vi "Halvorsen_Basic_Methods.vi"() -> ()   [LabVIEW 2016]
uses:
  <vilib>/Simulation/Scripting/Companion Diagram/SimConfigNode/SimParams.ctl
  <vilib>/Simulation/Scripting/Companion Diagram/SimConfigNode/_simSolvers.ctl
  <vilib>/Simulation/Implementation/Shared/SIMSCR Execution Mode.ctl
  <vilib>/Simulation/Param Hierarchy/Typedefs/SIMPH Param Control Actions.ctl
  <vilib>/Simulation/Implementation/Shared/SIM limit type.ctl
  <vilib>/Simulation/Implementation/Shared/NILVSim_ParamChanged.vi
  <vilib>/Simulation/Implementation/Shared/NILVSIM_BeginStep.vi
  <vilib>/Simulation/ContinuousLinear/Implementation/NILVSim Integrator new.llb/SIM Integrator Distributor (vector).vi
  <vilib>/Simulation/Utility/Implementation/NILVSim Collector.llb/SIM Collector (scalar).vi
  <vilib>/Simulation/ContinuousLinear/Implementation/NILVSim Integrator new.llb/SIM Integrator Collector (vector).vi
  <vilib>/Simulation/Implementation/Shared/NILVSim_Manager.vi
  <vilib>/Utility/error.llb/Clear Errors.vi
  <vilib>/Simulation/Implementation/Shared/NILVSim_FinalizeModel.vi
  <vilib>/Simulation/Utility/Implementation/NILVSim Collector.llb/NILVSim Collector core (scalar).vi
  <vilib>/Simulation/Implementation/Shared/SIM Unbundle Sim Info.vi
  <vilib>/Simulation/Implementation/Shared/NILVSim_Initialize.vi
  <vilib>/Simulation/Utility/Implementation/NILVSim Get Time and IsAcceptedStep.vi
  <vilib>/Simulation/Implementation/Shared/SIMSH Read Queue.vi
  <vilib>/Simulation/Implementation/Shared/NILVSim_GetModelError.vi
  <vilib>/Simulation/Implementation/Shared/SIM Bundle Sim Info.vi
  <vilib>/Simulation/Scripting/Companion Diagram/SimConfigNode/SimDog.xnode
  <vilib>/Simulation/Implementation/XNodeFramework/SimXNode/SimX.xnode
  <vilib>/Simulation/ContinuousLinear/Implementation/NILVSim Integrator new.llb/SIM Integrator (vector).vi
  <vilib>/Simulation/Implementation/Shared/NI_SIM_Implementation.lvlib
panel:
  in  "Method Stepsize":dbl=0.01
  in  "Parameters":dbl[](array[numeric])=[0.1, 0.1, 0.1]
  in  "Method":u16=1
  out "Абсолютная погрешность":ext[][](graph)
  out "last_point_Thomas":dbl[](array[numeric])=[2.5014012033767568, 0.2778214910167161, 0.25145974992803094] format="%#_22f"
  in  "ODE Solver":T1(ring)=enum."Runge-Kutta 45 (variable)"
  out "Временная область":dbl[][](graph)
  in  "SM Step":dbl=0.005
  in  "T":dbl=100.0
  in  "Intial condition":dbl[](array[knob])=[1.0, 0.0, 1.0] scale=-10.0..10.0
  # "0,19"
  # "0,1"
  # "0,208186"
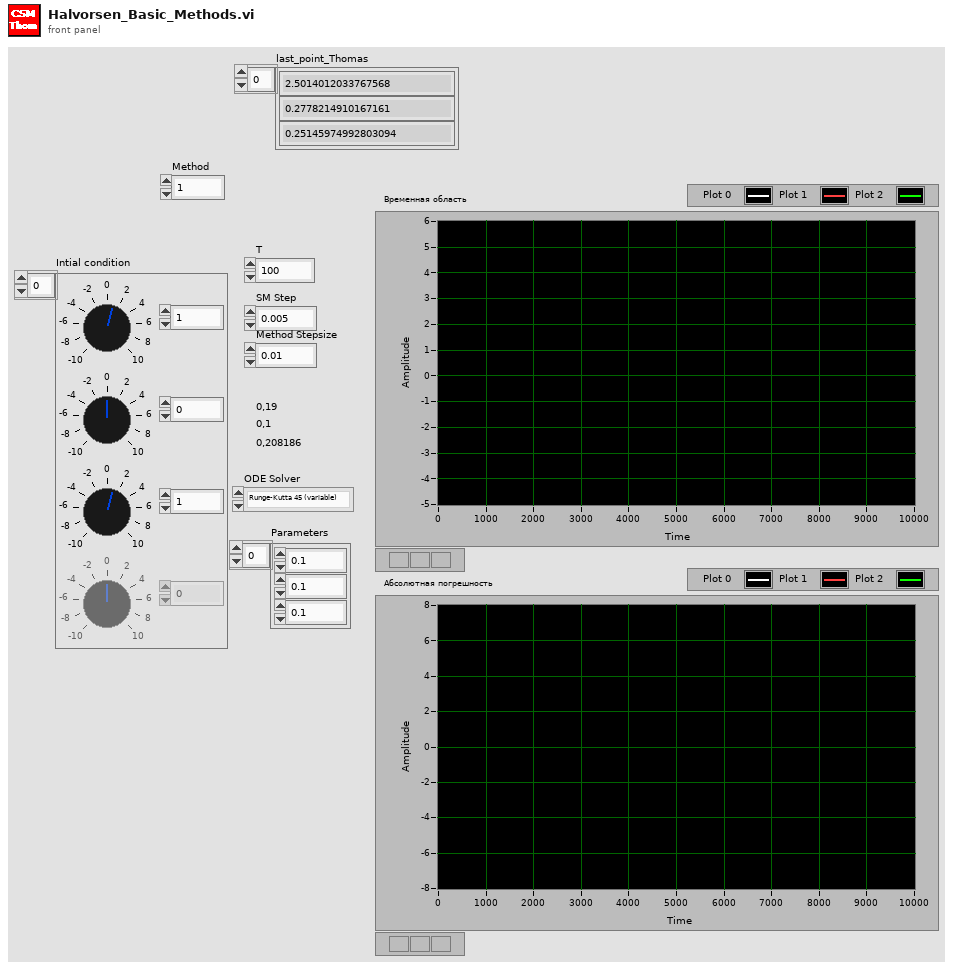
[diagram p1: front panel]
types:
  T1 = enum16{"Runge-Kutta 1 (Euler)", "Runge-Kutta 2", "Runge-Kutta 3", "Runge-Kutta 4", "Runge-Kutta 23 (variable)", "Runge-Kutta 45 (variable)", "BDF (variable)", "Adams-Moulton (variable)", "Rosenbrock (variable)", "Discrete States Only", "SDIRK 4 (variable)", "Radau 5 (variable)", "Radau 9 (variable)", "Radau 13 (variable)", "Radau [Variable Order] (variable)", "Gear's Method (variable)"}
  T2 = enum16{"Euler", "Cromer 1", "Cromer 2", "D1", "D2", "PD1", "PD2", "CD1", "CD2", "CD3", "CD4", "IMP", "LIMP", "IEuler", "SEMP", "SIMP", "EMP", "MEMP"}
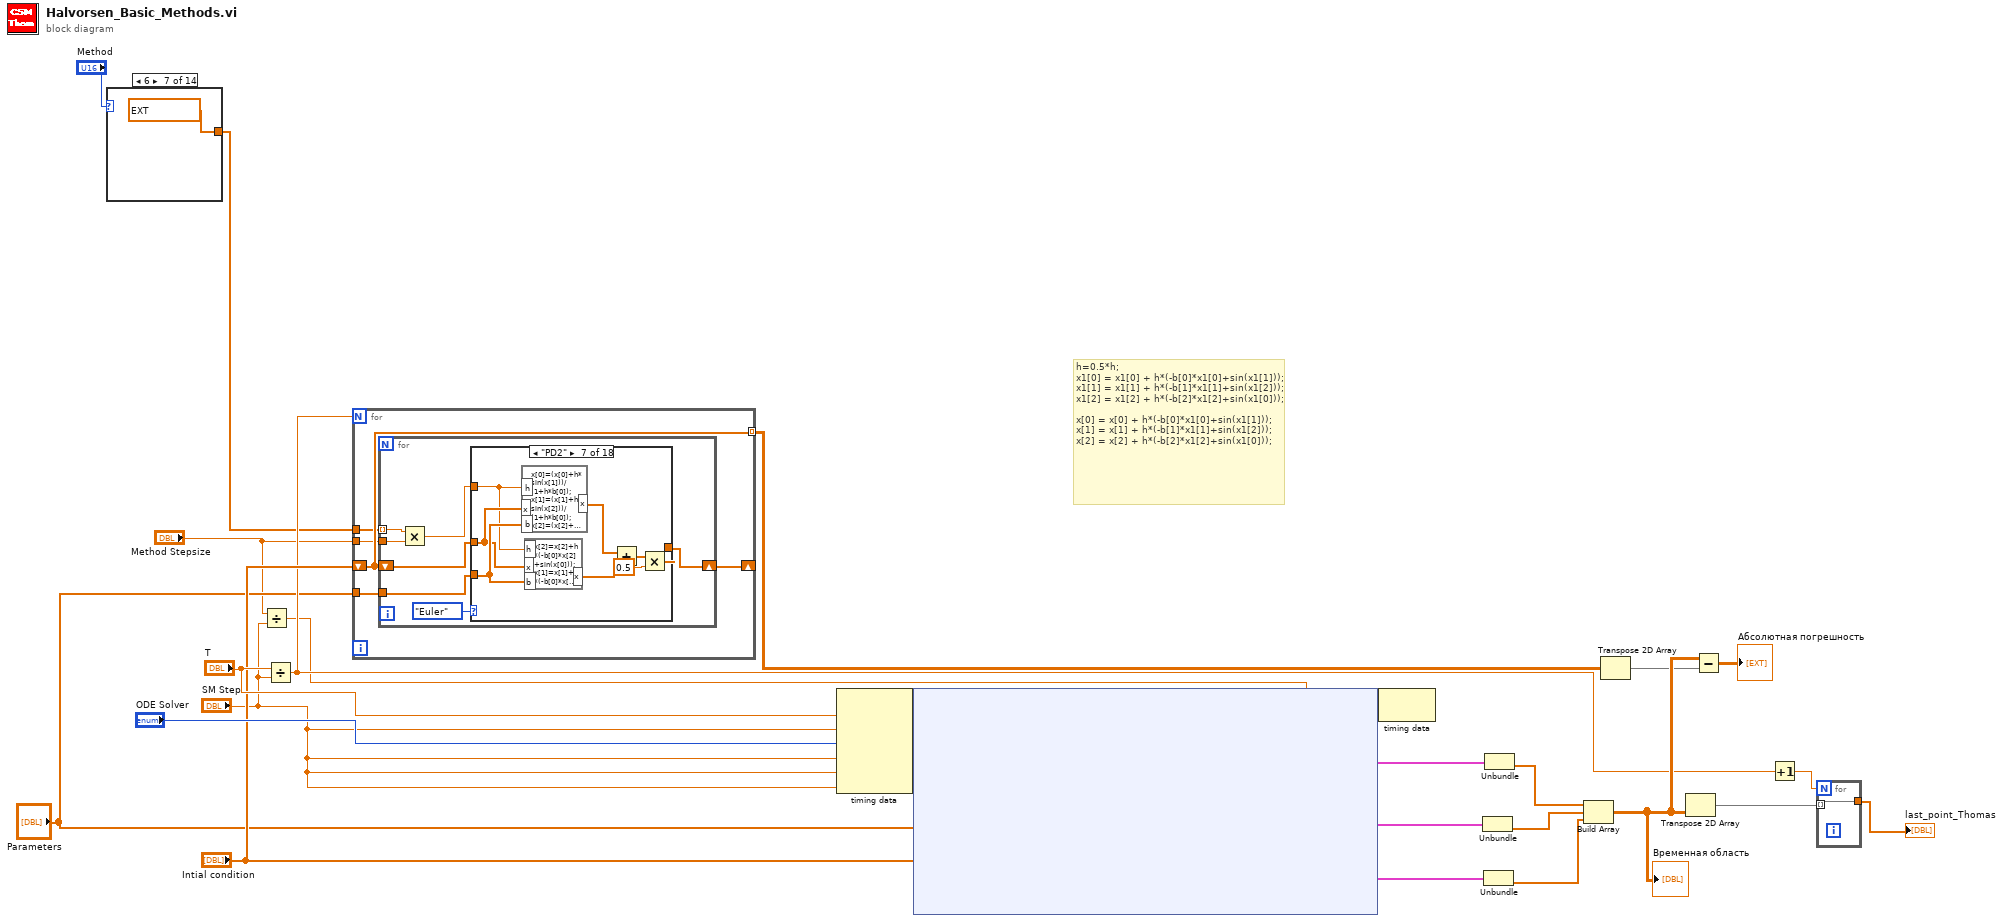
[diagram p0: block diagram]
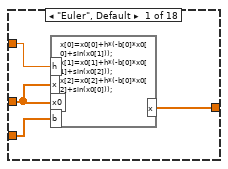
[diagram p2: hidden frame]
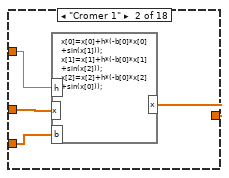
[diagram p3: hidden frame]
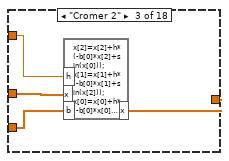
[diagram p4: hidden frame]
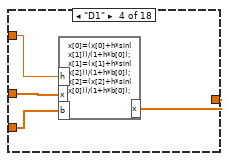
[diagram p5: hidden frame]
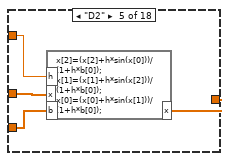
[diagram p6: hidden frame]
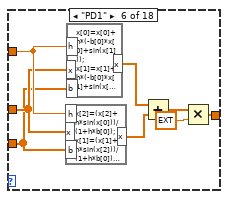
[diagram p7: hidden frame]
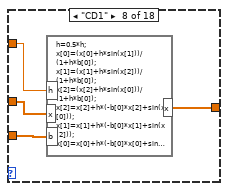
[diagram p8: hidden frame]
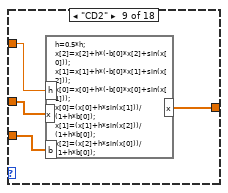
[diagram p9: hidden frame]
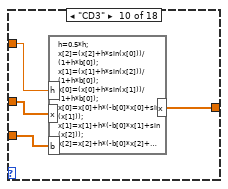
[diagram p10: hidden frame]
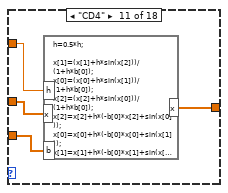
[diagram p11: hidden frame]
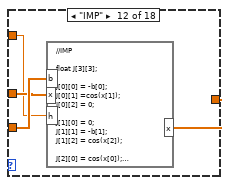
[diagram p12: hidden frame]
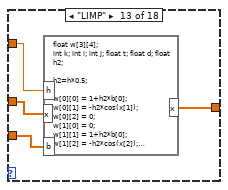
[diagram p13: hidden frame]
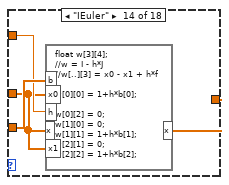
[diagram p14: hidden frame]
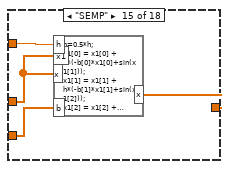
[diagram p15: hidden frame]
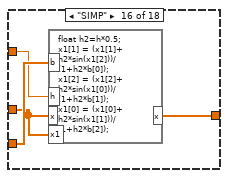
[diagram p16: hidden frame]
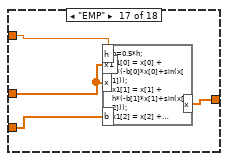
[diagram p17: hidden frame]
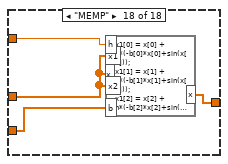
[diagram p18: hidden frame]
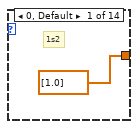
[diagram p19: hidden frame]
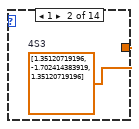
[diagram p20: hidden frame]
diagram:
  # "h=0.5*h;\nx1[0] = x1[0] + h*(-b[0]*x1[0]+sin(x1[1])); \nx1[1] = x1[1] + h*(-b[1]*x1[1]+sin(x1[2])); \nx1[2] = x1[2] + h*(-b[2]*x1[2]+sin(x1[0]));\n\nx[0] = x[0] + h*(-b[0]*x1[0]+sin(x1[1])); \nx[1] = x[1] + h*(-b[1]*x1[1]+sin(x1[2])); \nx[2] = x[2] + h*(-b[2]*x1[2]+sin(x1[0]));"
  n1 = case shown="6" "Method" {
    tunnel: [dbl[] [1.0] w27 ext[] [0.78451361047755726003, 0.23557321335935813, -1.17767998417887099995, 1.3151863206839112, -1.17767998417887099995, 0.23557321335935813, 0.78451361047755726003] ext[] [0.392161444007314139, 0.332599136789359438, -0.70624617255763935903, 0.082213596293550800203, 0.79854399093482996298, 0.082213596293550800203, -0.70624617255763935903, 0.332599136789359438, 0.392161444007314139] ext[] [0.391030203308684788, 0.334037289611136017, -0.706227281187561343, 0.0818775496480594457, 0.798564477239362184, 0.0818775496480594457, -0.706227281187561343, 0.334037289611136017, 0.391030203308684788] ext[] [0.741670364350612953, -0.409100825800031594, 0.190754710296238379, -0.573862471116082266, 0.299064181303655923, 0.334624918245298183, 0.315293092396766596, -0.79688793935291635402, 0.315293092396766596, 0.334624918245298183, 0.299064181303655923, -0.573862471116082266, 0.190754710296238379, -0.409100825800031594, 0.741670364350612953] ext[] [0.130202483088890080004, 0.561162981775108384, -0.389474962644847286, 0.15884190655515560001, -0.395903894133237577, 0.18453964097831570699, 0.258374387686322047, 0.295011723609310298, -0.605508533830034511, 0.295011723609310298, 0.258374387686322047, 0.18453964097831570699, -0.395903894133237577, 0.15884190655515560001, -0.389474962644847286, 0.561162981775108384, 0.130202483088890080004] ext[] [0.127136927734878578996, 0.56170253798880269902, -0.382534719948830188, 0.160076056294647430995, -0.401816374326806966, 0.187366716542278497, 0.26070870920779240501, 0.29039738812516162301, -0.60607448323584816197, 0.29039738812516162301, 0.26070870920779240501, 0.187366716542278497, -0.401816374326806966, 0.160076056294647430995, -0.382534719948830188, 0.56170253798880269902, 0.127136927734878578996] w34 ext[] [-0.481598956002530028, 0.00363039315445959268, 0.50180317558723140197, 0.282984026245062548, 0.807029678953722238, -0.0260905805385922054, -0.872865901463180715, -0.523735680625105816, 0.44521844299952789201, 0.18612289547097907799, 0.231373278664383606, -0.521910365904186289, 0.748661137144992967, 0.066736511890604057497, -0.80360324375670830302, 0.912490376358679945, -0.80360324375670830302, 0.066736511890604057497, 0.748661137144992967, -0.521910365904186289, 0.231373278664383606, 0.18612289547097907799, 0.44521844299952789201, -0.523735680625105816, -0.872865901463180715, -0.0260905805385922054, 0.807029678953722238, 0.282984026245062548, 0.50180317558723140197, 0.00363039315445959268, -0.481598956002530028] ext[] [0.27338476926228452699, 0.445878465025602839, 0.832196428471363071, -0.833968685549579428, 0.278918430570151942, 0.89032738045702531997, 0.0566815148452457094, -0.857374208149788877, -0.467894925548365861, -0.479190091823982642, 0.167240746800437089, -0.874431512633761433, -0.498734818536201657, 0.58930536608974918802, 0.834589377908827297, 0.28614352562198582699, 0.834589377908827297, 0.58930536608974918802, -0.498734818536201657, -0.874431512633761433, 0.167240746800437089, -0.479190091823982642, -0.467894925548365861, -0.857374208149788877, 0.0566815148452457094, 0.89032738045702531997, 0.278918430570151942, -0.833968685549579428, 0.832196428471363071, 0.445878465025602839, 0.27338476926228452699] ext[] [0.0704288776826580668, 0.87415651735353949, 0.0554146049638024427, -0.0668004778987970115, -0.626413089587995555, 0.236826210875287628, -0.422210634031700542, 0.242229422010408592, 0.047374515478601436501, 0.543868260524724233, -0.932522309284472643, 0.169601798836764648, 0.71608567578450563602, -0.80016730247310573502, 0.237781852922567707, -0.323303015508639433, 0.955298184703702076, -0.323303015508639433, 0.237781852922567707, -0.80016730247310573502, 0.71608567578450563602, 0.169601798836764648, -0.932522309284472643, 0.543868260524724233, 0.047374515478601436501, 0.242229422010408592, -0.422210634031700542, 0.236826210875287628, -0.626413089587995555, -0.0668004778987970115, 0.0554146049638024427, 0.87415651735353949, 0.0704288776826580668] ext[] [0.12282427644721572, 0.77644680890696440298, 0.148815145537342974, -0.172391259535060672, -0.547459957818524637, 0.145129323273069274, -0.315645551531144605, 0.120868650898338719, 0.179102775178663442, 0.442634088139932459, -0.819353374795936974, 0.13445474141752884001, 0.644442391690166465, -0.719301493702016125, 0.21036902497348664599, -0.26908194941570516201, 0.836292720671358462, -0.26908194941570516201, 0.21036902497348664599, -0.719301493702016125, 0.644442391690166465, 0.13445474141752884001, -0.819353374795936974, 0.442634088139932459, 0.179102775178663442, 0.120868650898338719, -0.315645551531144605, 0.145129323273069274, -0.547459957818524637, -0.172391259535060672, 0.148815145537342974, 0.77644680890696440298, 0.12282427644721572] ext[] [0.12313526870982994, 0.77644981696937310502, 0.149054900795670456, -0.17250761219393744401, -0.54871240818800177898, 0.142897654218418421, -0.314191932639868619, 0.12670943739561041, 0.17444734584181312899, 0.443185446654285729, -0.819489005682990844, 0.133825457384895829996, 0.64509023524410605, -0.719363371699220607, -0.719363371699220607, -0.26828113140636051899, 0.83647216092348048903, -0.26828113140636051899, -0.719363371699220607, -0.719363371699220607, 0.64509023524410605, 0.133825457384895829996, -0.819489005682990844, 0.443185446654285729, 0.17444734584181312899, 0.12670943739561041, -0.314191932639868619, 0.142897654218418421, -0.54871240818800177898, -0.17250761219393744401, 0.149054900795670456, 0.77644981696937310502, 0.12313526870982994]] -> w6
    frame 0, Default {
      # "1s2"
    }
    frame 1 {
      w27 = dbl[] [1.35120719196, -1.702414383919, 1.35120719196]  # 4S3
    }
    frame 2 {
      # "6s7"
    }
    frame 3 {
      # "6s9"
    }
    frame 4 {
    }
    frame 5 {
    }
    frame 6 {
    }
    frame 7 {
    }
    frame 8 {
      w34 = dbl[] [-0.48159895600253005, 0.0036303931544595927, 0.5018031755872314, 0.2829840262450625, 0.8070296789537222, -0.026090580538592204, -0.8728659014632, -0.5237356806251, 0.4452184429995, 0.186122895471, 0.2313732786644, -0.5219103659042, 0.748661137145, 0.0667365118906, -0.8036032437567, 0.9124903763587, -0.8036032437567, 0.06673651189060406, 0.7486611371449929, -0.5219103659041863, 0.23137327866438362, 0.18612289547097907, 0.4452184429995279, -0.5237356806251058, -0.8728659014631807, -0.026090580538592204, 0.8070296789537222, 0.2829840262450625, 0.5018031755872314, 0.0036303931544595927, -0.48159895600253005]  # 8s31
    }
    frame 9 {
    }
    frame 10 {
    }
    frame 11 {
    }
    frame 12 {
    }
    frame 13 {
    }
  }
  n2 = Divide(x="Method Stepsize", y="SM Step") -> (x/y=w1:dbl)
  n3 = Divide(x="T", y="SM Step") -> (x/y=w8:dbl)
  n4 = for {
    N: w8 -> [_]
    shift-right: [w44] -> _
    shift-left: "Intial condition" -> [w43]
    tunnel: "Parameters" -> [w40]
    tunnel: "Method Stepsize" -> [w41]
    tunnel: [w43] -> w5 mode=indexing
    tunnel: w6 -> [w42]
    n5 = for {
      shift-right: [w49] -> w44
      shift-left: w43 -> [w47]
      tunnel: w42 -> [w51] mode=indexing
      tunnel: w41 -> [w50]
      tunnel: w40 -> [w46]
      n6 = Multiply(x=w51, y=w50) -> (x*y=w48:ext)
      n7 = case shown="\"PD2\"" T2."Euler" ("Method") {
        tunnel: w48 -> [w53 w59 w62 w66 w71 w74 w80 w90 w94 w99 w102 w104 w111 w114 w118 w121 w125 w129]
        tunnel: w46 -> [w55 w57 w60 w64 w69 w72 w82 w88 w92 w97 w100 w106 w108 w115 w116 w122 w126 w130]
        tunnel: w47 -> [w54 w58 w61 w65 w70 w73 w81 w89 w93 w98 w101 w105 w109 w113 w117 w120 w124 w131]
        tunnel: [w52 w56 w63 w67 w68 w75 w83 w91 w95 w96 w103 w107 w110 w112 w119 w123 w127 w128] -> w49
        frame "Euler", Default {
          n8 = formula code="x[0]=x0[0]+h*(-b[0]*x0[0]+sin(x0[1]));\nx[1]=x0[1]+h*(-b[0]*x0[1]+sin(x0[2]));\nx[2]=x0[2]+h*(-b[0]*x0[2]+sin(x0[0]));"("x"=w54, "x0"=w54, "b"=w55, "h"=w53) -> ("x"=w52:ext[])
        }
        frame "Cromer 1" {
          n9 = formula code="x[0]=x[0]+h*(-b[0]*x[0]+sin(x[1]));\nx[1]=x[1]+h*(-b[0]*x[1]+sin(x[2]));\nx[2]=x[2]+h*(-b[0]*x[2]+sin(x[0]));"("x"=w58, "b"=w57, "h"=w59) -> ("x"=w56:ext[])
        }
        frame "Cromer 2" {
          n10 = formula code="x[2]=x[2]+h*(-b[0]*x[2]+sin(x[0]));\nx[1]=x[1]+h*(-b[0]*x[1]+sin(x[2]));\nx[0]=x[0]+h*(-b[0]*x[0]+sin(x[1]));"("x"=w61, "b"=w60, "h"=w62) -> ("x"=w63:ext[])
        }
        frame "D1" {
          n11 = formula code="x[0]=(x[0]+h*sin(x[1]))/(1+h*b[0]);\nx[1]=(x[1]+h*sin(x[2]))/(1+h*b[0]);\nx[2]=(x[2]+h*sin(x[0]))/(1+h*b[0]);"("x"=w65, "b"=w64, "h"=w66) -> ("x"=w67:ext[])
        }
        frame "D2" {
          n12 = formula code="x[2]=(x[2]+h*sin(x[0]))/(1+h*b[0]);\nx[1]=(x[1]+h*sin(x[2]))/(1+h*b[0]);\nx[0]=(x[0]+h*sin(x[1]))/(1+h*b[0]);"("x"=w70, "b"=w69, "h"=w71) -> ("x"=w68:ext[])
        }
        frame "PD1" {
          n13 = formula code="x[2]=(x[2]+h*sin(x[0]))/(1+h*b[0]);\nx[1]=(x[1]+h*sin(x[2]))/(1+h*b[0]);\nx[0]=(x[0]+h*sin(x[1]))/(1+h*b[0]);"("x"=w73, "b"=w72, "h"=w74) -> ("x"=w77:ext[])
          n14 = formula code="x[0]=x[0]+h*(-b[0]*x[0]+sin(x[1]));\nx[1]=x[1]+h*(-b[0]*x[1]+sin(x[2]));\nx[2]=x[2]+h*(-b[0]*x[2]+sin(x[0]));"("x"=w73, "b"=w72, "h"=w74) -> ("x"=w76:ext[])
          n15 = Add(x=w76, y=w77) -> (x+y=w78:ext[])
          n16 = Multiply(x=w78, y=ext 0.5) -> (x*y=w75:ext[])
        }
        frame "PD2" {
          n17 = formula code="x[0]=(x[0]+h*sin(x[1]))/(1+h*b[0]);\nx[1]=(x[1]+h*sin(x[2]))/(1+h*b[0]);\nx[2]=(x[2]+h*sin(x[0]))/(1+h*b[0]);"("x"=w81, "b"=w82, "h"=w80) -> ("x"=w87:ext[])
          n18 = formula code="x[2]=x[2]+h*(-b[0]*x[2]+sin(x[0]));\nx[1]=x[1]+h*(-b[0]*x[1]+sin(x[2]));\nx[0]=x[0]+h*(-b[0]*x[0]+sin(x[1]));"("x"=w81, "b"=w82, "h"=w80) -> ("x"=w86:ext[])
          n19 = Add(x=w87, y=w86) -> (x+y=w85:ext[])
          n20 = Multiply(x=w85, y=0.5) -> (x*y=w83:ext[])
        }
        frame "CD1" {
          n21 = formula code="h=0.5*h;\nx[0]=(x[0]+h*sin(x[1]))/(1+h*b[0]);\nx[1]=(x[1]+h*sin(x[2]))/(1+h*b[0]);\nx[2]=(x[2]+h*sin(x[0]))/(1+h*b[0]);\nx[2]=x[2]+h*(-b[0]*x[2]+sin(x[0]));\nx[1]=x[1]+h*(-b[0]*x[1]+sin(x[2]));\nx[0]=x[0]+h*(-b[0]*x[0]+sin(x[1]));"("x"=w89, "b"=w88, "h"=w90) -> ("x"=w91:ext[])
        }
        frame "CD2" {
          n22 = formula code="h=0.5*h;\nx[2]=x[2]+h*(-b[0]*x[2]+sin(x[0]));\nx[1]=x[1]+h*(-b[0]*x[1]+sin(x[2]));\nx[0]=x[0]+h*(-b[0]*x[0]+sin(x[1]));\nx[0]=(x[0]+h*sin(x[1]))/(1+h*b[0]);\nx[1]=(x[1]+h*sin(x[2]))/(1+h*b[0]);\nx[2]=(x[2]+h*sin(x[0]))/(1+h*b[0]);"("x"=w93, "b"=w92, "h"=w94) -> ("x"=w95:ext[])
        }
        frame "CD3" {
          n23 = formula code="h=0.5*h;\nx[2]=(x[2]+h*sin(x[0]))/(1+h*b[0]);\nx[1]=(x[1]+h*sin(x[2]))/(1+h*b[0]);\nx[0]=(x[0]+h*sin(x[1]))/(1+h*b[0]);\nx[0]=x[0]+h*(-b[0]*x[0]+sin(x[1]));\nx[1]=x[1]+h*(-b[0]*x[1]+sin(x[2]));\nx[2]=x[2]+h*(-b[0]*x[2]+sin(x[0]));"("x"=w98, "b"=w97, "h"=w99) -> ("x"=w96:ext[])
        }
        frame "CD4" {
          n24 = formula code="h=0.5*h;\n\nx[1]=(x[1]+h*sin(x[2]))/(1+h*b[0]);\nx[0]=(x[0]+h*sin(x[1]))/(1+h*b[0]);\nx[2]=(x[2]+h*sin(x[0]))/(1+h*b[0]);\nx[2]=x[2]+h*(-b[0]*x[2]+sin(x[0]));\nx[0]=x[0]+h*(-b[0]*x[0]+sin(x[1]));\nx[1]=x[1]+h*(-b[0]*x[1]+sin(x[2]));"("x"=w101, "b"=w100, "h"=w102) -> ("x"=w103:ext[])
        }
        frame "IMP" {
          n25 = formula code="//IMP\n\nfloat J[3][3];\n\nJ[0][0] = -b[0]; \nJ[0][1] =cos(x[1]); \nJ[0][2] = 0; \n\nJ[1][0] = 0; \nJ[1][1] = -b[1];\nJ[1][2] = cos(x[2]);\n\nJ[2][0] = cos(x[0]); \nJ[2][1] =0;\nJ[2][2] = -b[2];\n\n\nfloat w[3][4], Z[3], a[3], Zn[3], dz;\nfloat tol;\nint k; int i; int j; float t; float d;\ntol = 1e-14;\nint nnewtmax = 3, nnewt;\ndz = 2e-13;\nnnewt = 0;\n\nZ[0] = x[0]; Z[1] = x[1]; Z[2] = x[2];\nwhile ( (dz > tol) && (nnewt < nnewtmax)){\n\nfor(i=0;i<3;i++){\nfor(j=0;j<3;j++){\nif (i==j)\nw[i][j]=1 - 0.5*h*J[i][j];\nelse\nw[i][j]= - 0.5*h*J[i][j];\n}}\n\n\n\na[0] = 0.5*(x[0] + Z[0]);\na[1] = 0.5*(x[1] + Z[1]);\na[2] = 0.5*(x[2] + Z[2]);\n\n\n\nw[0][3]=-Z[0]+x[0]+h*(-b[0]*a[0]+sin(a[1]));\nw[1][3]= -Z[1]+x[1]+h*(-b[1]*a[1]+sin(a[2]));\nw[2][3]= -Z[2]+x[2]+h*(-b[2]*a[2]+sin(a[0]));\n\n\nfor(k = 0; k <= 1; k++){\n\tint l = k;\n\n\tfor( i = k+1; i<= 2; i++){\n\t\tif( abs(w[i][k]) > abs(w[l][k]) ){\n\t\t\tl = i;\n\t\t}\n\t}\n\tif (l != k){\n\t\tfor( j = 0; j <= 3; j++){\n\t\t\tif ((j == 0) || (j >= k)){\n\t\t\t\tt = w[k][j];\n\t\t\t\tw[k][j] = w[l][j];\n\t\t\t\tw[l][j] = t;\n\t\t\t}\n\t\t}\n\t}\t\n\n\td = 1.0 / w[k][k];\n\tfor( i=(k+1); i <=(2); i++){\n\t\tif (w[i][k] == 0){\n\t\t\tcontinue;\n\t\t}\n\t\tt = w[i][k] * d;\n\t\tfor ( j = k; j <= (3); j++) {\n\t\t\tif (w[k][j] != 0){\n\t\t\t\tw[i][j] = w[i][j] - t * w[k][j];\n\t\t\t}\n\t\t}\n\t}\n}\nfor( i=(3); i >= 2; i--){\n\tfor( j=1; j <= i-1; j++){\n\t\tt = w[i - j - 1][i - 1]/w[ i -1][i - 1];\n\t\tw[i-j - 1][ 3] = w[i-j -1][3] - t*w[i - 1][ 3];\n\t}\n\tw[i-1][ 3] = w[i - 1][3]/w[ i -1][i - 1];\n}\nw[0][3] = w[0][3]/w[0][0];\nZn[0] = Z[0]+ w[0][3];\nZn[1] = Z[1]+ w[1][3];\nZn[2] = Z[2]+ w[2][3];\n\ndz = ( (Zn[0] - Z[0])**2 + (Zn[1] - Z[1])**2 + (Zn[2] - Z[2])**2 )**0.5;\nZ[0] = Zn[0];\nZ[1] = Zn[1];\nZ[2] = Zn[2];\n\n\nnnewt ++;\n}\n\nx[0] = Zn[0];\nx[1] = Zn[1];\nx[2] = Zn[2];"("x"=w105, "h"=w104, "b"=w106) -> ("x"=w107:ext[])
        }
        frame "LIMP" {
          n26 = formula code="float w[3][4];\nint k; int i; int j; float t; float d; float h2;\n\nh2=h*0.5;\n\nw[0][0] = 1+h2*b[0];\nw[0][1] = -h2*cos(x[1]);\nw[0][2] = 0;\nw[1][0] = 0;\nw[1][1] = 1+h2*b[0];\nw[1][2] = -h2*cos(x[2]);\nw[2][0] = -h2*cos(x[0]);\nw[2][1] = 0;\nw[2][2] = 1+h2*b[0];\n\nw[0][3] = h*(-b[0]*x[0]+sin(x[1]));\nw[1][3] = h*(-b[0]*x[1]+sin(x[2]));\nw[2][3] = h*(-b[0]*x[2]+sin(x[0]));\n\nint HEIGHT = 3;\nint  WIDTH = 4;\nfor(k = 0; k <= HEIGHT-2; k++){\n\nint\tl = k;\n\nfor( i = k+1;  i<= HEIGHT-1; i++){\n\t\t\tif( abs(w[i][k]) > abs(w[l][k]) ){\n\t\t\t\tl = i;\n    }\n   }\n\t\tif (l != k){\n\t\t\tfor( j = 0; j <= WIDTH-1; j++){\n\t\t\t\tif ((j == 0) || (j >= k)){\n\t\t\t\t\tt = w[k][j];\n\t\t\t\t\tw[k][j] = w[l][j];\n\t\t\t\t\tw[l][j] = t;\n                }\n            }\n        }\n\n\t\td = 1.0 / w[k][k];\n\t\tfor( i=(k+1); i <=(HEIGHT-1); i++){\n\t\t\tif (w[i][k] == 0){\n                continue;\n            }\n\t\t\tt = w[i][k] * d;\n\t\t\tfor ( j = k; j <= (WIDTH-1); j++) {\n\t\t\t\tif (w[k][j] != 0){\n\t\t\t\t\tw[i][j] = w[i][j] - t * w[k][j];\n                }\n            }\n        }\n    }\n    \n\t\n    for( i=(HEIGHT); i >= 2; i--){ \n        for( j=1; j <= i-1; j++){\n            t = w[i - j - 1][i - 1]/w[ i -1][i - 1];\n            w[i-j - 1][ WIDTH- 1] = w[i-j -1][ WIDTH -1] - t*w[i - 1][ WIDTH -1];\n        }\n        w[i-1][ WIDTH-1] = w[i - 1][ WIDTH - 1]/w[ i -1][i - 1];\n    }\n    w[0][ WIDTH - 1] = w[0][ WIDTH -1]/w[0][0];\n\n    \n    x[0] =x[0]+ w[0][WIDTH - 1];\n    x[1] = x[1]+w[1][WIDTH - 1];\n    x[2] = x[2]+w[2][WIDTH - 1];"("x"=w109, "b"=w108, "h"=w111) -> ("x"=w110:ext[])
        }
        frame "IEuler" {
          n27 = formula code="float w[3][4];\n//w = I - h*J\n//w[..][3] = x0 - x1 + h*f\n\nw[0][0] = 1+h*b[0];\n\nw[0][2] = 0;\nw[1][0] = 0;\nw[1][1] = 1+h*b[1];\nw[2][1] = 0;\nw[2][2] = 1+h*b[2];\n\n\n\nfloat tol = 1e-12;\nfloat dx = 2*tol;\n\nint nmax = 10;\nint n = 0;\n//цикл по Ньютонам\nwhile ((dx > tol)&&(n < nmax)){\n\nw[0][1] = -h*cos(x[1]);\nw[1][2] = -h*cos(x[2]);\nw[2][0] = -h*cos(x[0]);\n\nw[0][3] = x0[0] - x1[0] +  h*(-b[0]*x[0]+sin(x[1]));\nw[1][3] = x0[1] - x1[1] + h*(-b[1]*x[1]+sin(x[2]));\nw[2][3] = x0[2] - x1[2] + h*(-b[2]*x[2]+sin(x[0]));\n\nint HEIGHT = 3;\nint  WIDTH = 4;\nint k; int i; int j; float t; float d;\n\nfor(k = 0; k <= HEIGHT-2; k++){\n\tint\tl = k;\n\tfor( i = k+1;  i<= HEIGHT-1; i++){\n\t\t\t\tif( abs(w[i][k]) > abs(w[l][k]) ){\n\t\t\t\t\tl = i;\n\t\t}\n   }\n\t\tif (l != k){\n\t\t\tfor( j = 0; j <= WIDTH-1; j++){\n\t\t\t\tif ((j == 0) || (j >= k)){\n\t\t\t\t\tt = w[k][j];\n\t\t\t\t\tw[k][j] = w[l][j];\n\t\t\t\t\tw[l][j] = t;\n                }\n            }\n        }\n\t\t\n\t\td = 1.0 / w[k][k];\n\t\tfor( i=(k+1); i <=(HEIGHT-1); i++){\n\t\t\tif (w[i][k] == 0){\n                continue;\n            }\n\t\t\tt = w[i][k] * d;\n\t\t\tfor ( j = k; j <= (WIDTH-1); j++) {\n\t\t\t\tif (w[k][j] != 0){\n\t\t\t\t\tw[i][j] = w[i][j] - t * w[k][j];\n                }\n            }\n        }\n    }\n\n    for( i=(HEIGHT); i >= 2; i--){ \n        for( j=1; j <= i-1; j++){\n            t = w[i - j - 1][i - 1]/w[ i -1][i - 1];\n            w[i-j - 1][ WIDTH- 1] = w[i-j -1][ WIDTH -1] - t*w[i - 1][ WIDTH -1];\n        }\n        w[i-1][ WIDTH-1] = w[i - 1][ WIDTH - 1]/w[ i -1][i - 1];\n    }\n    w[0][ WIDTH - 1] = w[0][ WIDTH -1]/w[0][0];\n\n    \n    x1[0] =x[0]+ w[0][WIDTH - 1];\n    x1[1] = x[1]+w[1][WIDTH - 1];\n    x1[2] = x[2]+w[2][WIDTH - 1];\n\ndx = sqrt((x1[0] - x[0])**2 + (x1[1] - x[1])**2 + (x1[2] - x[2])**2);\nn++;\n\nx[0] = x1[0]; x[1] = x1[1]; x[2] = x1[2];\n\n}"("x"=w113, "h"=w114, "x1"=w113, "b"=w115, "x0"=w113) -> ("x"=w112:ext[])
        }
        frame "SEMP" {
          n28 = formula code="h=0.5*h;\nx1[0] = x1[0] + h*(-b[0]*x1[0]+sin(x1[1])); \nx1[1] = x1[1] + h*(-b[1]*x1[1]+sin(x1[2])); \nx1[2] = x1[2] + h*(-b[2]*x1[2]+sin(x1[0]));\n\nx[0] = x[0] + h*(-b[0]*x1[0]+sin(x1[1])); \nx[1] = x[1] + h*(-b[1]*x1[1]+sin(x1[2])); \nx[2] = x[2] + h*(-b[2]*x1[2]+sin(x1[0]));"("x"=w117, "x1"=w117, "h"=w118, "b"=w116) -> ("x"=w119:ext[])
        }
        frame "SIMP" {
          n29 = formula code="float h2=h*0.5;\nx1[1] = (x1[1]+ h2*sin(x1[2]))/(1+h2*b[0]);\nx1[2] = (x1[2]+ h2*sin(x1[0]))/(1+h2*b[1]);\nx1[0] = (x1[0]+ h2*sin(x1[1]))/(1+h2*b[2]);\n\n\nx[0] = x[0] + h*(-b[0]*x1[0]+sin(x1[1]));\nx[1] = x[1] + h*(-b[1]*x1[1]+sin(x1[2]));\nx[2] = x[2] + h*(-b[2]*x1[2]+sin(x1[0]));"("x"=w120, "h"=w121, "x1"=w120, "b"=w122) -> ("x"=w123:ext[])
        }
        frame "EMP" {
          n30 = formula code="h=0.5*h;\nx1[0] = x[0] + h*(-b[0]*x[0]+sin(x[1])); \nx1[1] = x[1] + h*(-b[1]*x[1]+sin(x[2])); \nx1[2] = x[2] + h*(-b[2]*x[2]+sin(x[0]));\n\nx[0] = x[0] + h*(-b[0]*x1[0]+sin(x1[1])); \nx[1] = x[1] + h*(-b[1]*x1[1]+sin(x1[2])); \nx[2] = x[2] + h*(-b[2]*x1[2]+sin(x1[0]));"("x"=w124, "x1"=w124, "h"=w125, "b"=w126) -> ("x"=w127:ext[])
        }
        frame "MEMP" {
          n31 = formula code="x1[0] = x[0] + h*(-b[0]*x[0]+sin(x[1])); \nx1[1] = x[1] + h*(-b[1]*x[1]+sin(x[2])); \nx1[2] = x[2] + h*(-b[2]*x[2]+sin(x[0]));\nh=2*h;\n\nx2[0] = x[0] + h*(-b[0]*x1[0]+sin(x1[1])); \nx2[1] = x[1] + h*(-b[1]*x1[1]+sin(x1[2])); \nx2[2] = x[2] + h*(-b[2]*x1[2]+sin(x1[0]));\n\nx[0]=x1[0];\nx[1]=x1[1];\nx[2]=x1[2];\nx1[0]=x2[0];\nx1[1]=x2[1];\nx1[2]=x2[2];\nh=h*0.5;\nx2[0]=(x[0]+x1[0]+h*(-b[0]*x1[0]+sin(x1[1])))/2;\nx2[1]=(x[1]+x1[1]+h*(-b[1]*x1[1]+sin(x1[2])))/2;\nx2[2]=(x[2]+x1[2]+h*(-b[2]*x1[2]+sin(x1[0])))/2;"("x"=w131, "x1"=w131, "h"=w129, "b"=w130, "x2"=w131) -> ("x"=w128:ext[])
        }
      }
    }
  }
  n32 = node-c288("T", "SM Step", "ODE Solver", "SM Step", "SM Step", "SM Step") -> (w25:variant)
  n33 = node-c254 ("Control & Simulation Loop")(w25, "Parameters", "Intial condition", w1) -> (w24:variant, w23:cluster{"Time":dbl[], "Signal":dbl[]}, w22:cluster{"Time":dbl[], "Signal":dbl[]}, w21:cluster{"Time":dbl[], "Signal":dbl[]})
  n34 = node-c288(w24) -> ()  [unwired: 1 out]
  n35 = Unbundle(w22) -> ("Signal"=w19:dbl[])  [unwired: 1 out]
  n36 = Unbundle(w21) -> ("Signal"=w18:dbl[])  [unwired: 1 out]
  n37 = Unbundle(w23) -> ("Signal"=w20:dbl[])  [unwired: 1 out]
  n38 = Build Array(w20, w19, w18) -> (w12:dbl[][])
  "Временная область" <- w12
  n39 = Transpose 2D Array(2D array=w5) -> (transposed array=w11:ext[][])
  n40 = Transpose 2D Array(2D array=w12) -> (transposed array=w13:dbl[][])
  n41 = Subtract(x=w12, y=w11) -> (x-y=→"Абсолютная погрешность":ext[][])
  n42 = Increment(x=w8) -> (x+1=w16:dbl)
  n43 = for {
    N: w16 -> [_]
    tunnel: [w132] -> w14
    tunnel: w13 -> [w132] mode=indexing
  }
  "last_point_Thomas" <- w14
